vi "Autonomous Trajectories.vi"() -> ()   [LabVIEW 2015]
panel:
  out "3 Middle":T1(array[cluster])
  out "Go to Middle Goal":T1(array[cluster])
  out "Backward Pickup":T1(array[cluster])
  out "Forward Move Weight":T1(array[cluster])
  out "3 Right To High":T1(array[cluster])
  out "3 Left To High":T1(array[cluster])
  out "3 Descend Ramp":T1(array[cluster])
  out "3 Ascend Ramp":T1(array[cluster])
  out "Right One Go To High":T1(array[cluster])
  out "Left One Go To High":T1(array[cluster])
  out "One Back For Pickup":T1(array[cluster])
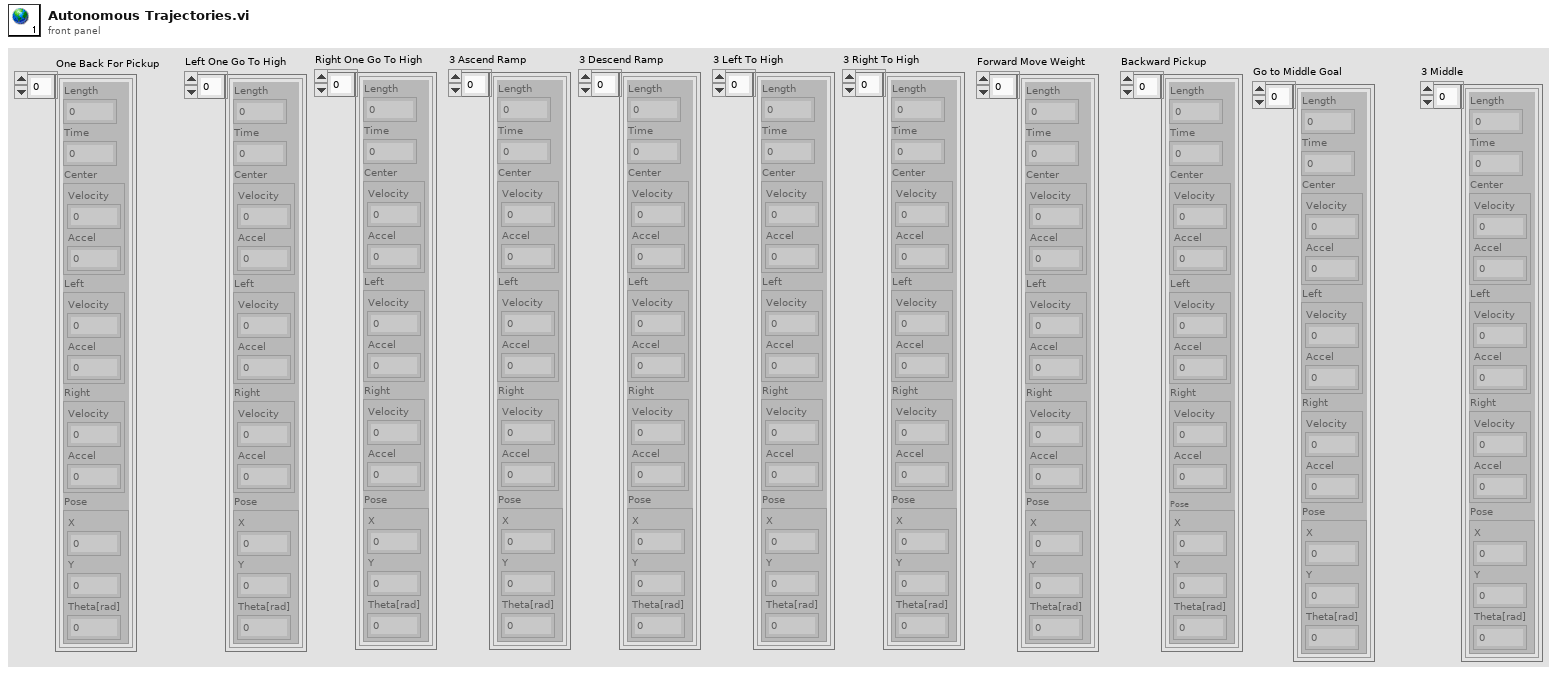
[diagram p1: front panel]
types:
  T1 = cluster{"Length":dbl, "Time":dbl, "Center":cluster{"Velocity":dbl, "Accel":dbl}, "Left":cluster{"Velocity":dbl, "Accel":dbl}, "Right":cluster{"Velocity":dbl, "Accel":dbl}, "Pose":cluster{"X":dbl, "Y":dbl, "Theta[rad]":dbl}}[]
diagram:
